vi "Tabelle auffeullen.vi"(8 "String":string="----", 11 "Neue Tabelle":T1) -> (3 "Tabelle":string[][](array[string]))   [LabVIEW 2020, in "Linearisierung v2.lvlib"]
uses:
  Linearisierung v2.lvlib
  Eingabetabelle.ctl
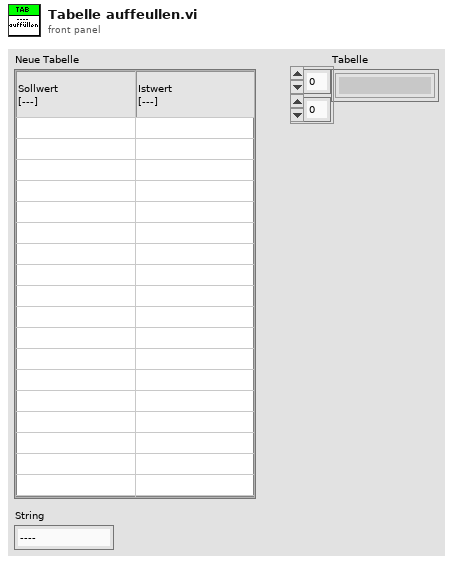
[diagram p1: front panel]
types:
  T1 = typedef "Linearisierung v2.lvlib/Eingabetabelle.ctl" = string[][]
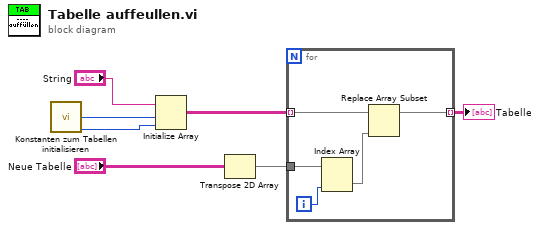
[diagram p0: block diagram]
diagram:
  n1 = call "Konstanten zum Tabellen initialisieren.vi"() -> ("Anzahl Tabellenzeilen"=w3:i32, "Anzahl Tabellenspalten"=w2:i32)  [unwired: 13 in, 1 out]
  n2 = Initialize Array("String", w3, w2) -> (w5:string[][])
  n3 = Transpose 2D Array(2D array="Neue Tabelle") -> (transposed array=w7:T1)
  n4 = for {
    tunnel: w5 -> [w12] mode=indexing
    tunnel: w7 -> [w11]
    tunnel: [w8] -> w4 mode=indexing
    i -> [w10]
    n5 = Index Array(array=w11, index (col)=w10) -> (element=w9:string[])  [unwired: 1 in]
    n6 = Replace Array Subset(array=w12, new element=w9) -> (w8:string[])  [unwired: 1 in]
  }
  "Tabelle" <- w4
